vi "nanocal -- nuclear schottky fit -- 2x2 -- V9.vi"() -> ()   [LabVIEW 2021] (continued)
0.149623565609 ,     0.141877858801 } , \r{    0.018836490895 ,     0.149623565609 ,     0.115522422306 } , \r{    0.022387211386 ,     0.149623565609 ,     0.093179863408 } , \r{    0.026607250598 ,     0.149623565609 ,     0.074729843493 } , \r{    0.031622776602 ,     0.149623565609 ,     0.059995877610 } , \r{    0.037583740429 ,     0.149623565609 ,     0.048775938318 } , \r{    0.044668359215 ,     0.149623565609 ,     0.040874020839 } , \r{    0.053088444423 ,     0.149623565609 ,     0.036127045463 } , \r{    0.063095734448 ,     0.149623565609 ,     0.034421884157 } , \r{    0.074989420933 ,     0.149623565609 ,     0.035699674200 } , \r{    0.089125093813 ,     0.149623565609 ,     0.039947569357 } , \r{    0.105925372518 ,     0.149623565609 ,     0.047180252600 } , \r{    0.125892541179 ,     0.149623565609 ,     0.057414385167 } , \r{    0.149623565609 ,     0.149623565609 ,     0.070639278795 } , \r{    0.177827941004 ,     0.149623565609 ,     0.086787357406 } , \r{    0.211348903984 ,     0.149623565609 ,     0.105708646760 } , \r{    0.251188643151 ,     0.149623565609 ,     0.127153912456 } , \r{    0.298538261892 ,     0.149623565609 ,     0.150770299518 } , \r{    0.354813389234 ,     0.149623565609 ,     0.176111225707 } , \r{    0.421696503429 ,     0.149623565609 ,     0.202659475022 } , \r{    0.501187233627 ,     0.149623565609 ,     0.229859851640 } , \r{    0.595662143529 ,     0.149623565609 ,     0.257156086913 } , \r{    0.707945784384 ,     0.149623565609 ,     0.284026281992 } , \r{    0.841395141645 ,     0.149623565609 ,     0.310012042831 } , \r{    0.001000000000 ,     0.177827941004 ,     0.740836835011 } , \r{    0.001188502227 ,     0.177827941004 ,     0.710329495354 } , \r{    0.001412537545 ,     0.177827941004 ,     0.677050447028 } , \r{    0.001678804018 ,     0.177827941004 ,     0.641106189632 } , \r{    0.001995262315 ,     0.177827941004 ,     0.602678568915 } , \r{    0.002371373706 ,     0.177827941004 ,     0.562039454503 } , \r{    0.002818382931 ,     0.177827941004 ,     0.519566808327 } , \r{    0.003349654392 ,     0.177827941004 ,     0.475755530109 } , \r{    0.003981071706 ,     0.177827941004 ,     0.431214355020 } , \r{    0.004731512590 ,     0.177827941004 ,     0.386642000254 } , \r{    0.005623413252 ,     0.177827941004 ,     0.342782601520 } , \r{    0.006683439176 ,     0.177827941004 ,     0.300369479723 } , \r{    0.007943282347 ,     0.177827941004 ,     0.260071698430 } , \r{    0.009440608763 ,     0.177827941004 ,     0.222455656817 } , \r{    0.011220184543 ,     0.177827941004 ,     0.187965930155 } , \r{    0.013335214322 ,     0.177827941004 ,     0.156921789373 } , \r{    0.015848931925 ,     0.177827941004 ,     0.129522861582 } , \r{    0.018836490895 ,     0.177827941004 ,     0.105859097961 } , \r{    0.022387211386 ,     0.177827941004 ,     0.085923590392 } , \r{    0.026607250598 ,     0.177827941004 ,     0.069629182896 } , \r{    0.031622776602 ,     0.177827941004 ,     0.056830202835 } , \r{    0.037583740429 ,     0.177827941004 ,     0.047349108968 } , \r{    0.044668359215 ,     0.177827941004 ,     0.041005320854 } , \r{    0.053088444423 ,     0.177827941004 ,     0.037641414898 } , \r{    0.063095734448 ,     0.177827941004 ,     0.037141549042 } , \r{    0.074989420933 ,     0.177827941004 ,     0.039438657457 } , \r{    0.089125093813 ,     0.177827941004 ,     0.044509677824 } , \r{    0.105925372518 ,     0.177827941004 ,     0.052360451062 } , \r{    0.125892541179 ,     0.177827941004 ,     0.063003162991 } , \r{    0.149623565609 ,     0.177827941004 ,     0.076429499384 } , \r{    0.177827941004 ,     0.177827941004 ,     0.092582860491 } , \r{    0.211348903984 ,     0.177827941004 ,     0.111333482638 } , \r{    0.251188643151 ,     0.177827941004 ,     0.132460756805 } , \r{    0.298538261892 ,     0.177827941004 ,     0.155646612919 } , \r{    0.354813389234 ,     0.177827941004 ,     0.180482156819 } , \r{    0.421696503429 ,     0.177827941004 ,     0.206487187930 } , \r{    0.501187233627 ,     0.177827941004 ,     0.233139638088 } , \r{    0.595662143529 ,     0.177827941004 ,     0.259910134828 } , \r{    0.707945784384 ,     0.177827941004 ,     0.286296242008 } , \r{    0.841395141645 ,     0.177827941004 ,     0.311851541843 } , \r{    0.001000000000 ,     0.211348903984 ,     0.658706462723 } , \r{    0.001188502227 ,     0.211348903984 ,     0.632229697281 } , \r{    0.001412537545 ,     0.211348903984 ,     0.603327363418 } , \r{    0.001678804018 ,     0.211348903984 ,     0.572087346120 } , \r{    0.001995262315 ,     0.211348903984 ,     0.538656633281 } , \r{    0.002371373706 ,     0.211348903984 ,     0.503252529375 } , \r{    0.002818382931 ,     0.211348903984 ,     0.466177332768 } , \r{    0.003349654392 ,     0.211348903984 ,     0.427831696047 } , \r{    0.003981071706 ,     0.211348903984 ,     0.388719014145 } , \r{    0.004731512590 ,     0.211348903984 ,     0.349433142339 } , \r{    0.005623413252 ,     0.211348903984 ,     0.310626218644 } , \r{    0.006683439176 ,     0.211348903984 ,     0.272961381709 } , \r{    0.007943282347 ,     0.211348903984 ,     0.237062250981 } , \r{    0.009440608763 ,     0.211348903984 ,     0.203472092487 } , \r{    0.011220184543 ,     0.211348903984 ,     0.172629846218 } , \r{    0.013335214322 ,     0.211348903984 ,     0.144862225297 } , \r{    0.015848931925 ,     0.211348903984 ,     0.120386368340 } , \r{    0.018836490895 ,     0.211348903984 ,     0.099317684423 } , \r{    0.022387211386 ,     0.211348903984 ,     0.081680417039 } , \r{    0.026607250598 ,     0.211348903984 ,     0.067421184763 } , \r{    0.031622776602 ,     0.211348903984 ,     0.056426796441 } , \r{    0.037583740429 ,     0.211348903984 ,     0.048546798094 } , \r{    0.044668359215 ,     0.211348903984 ,     0.043619100040 } , \r{    0.053088444423 ,     0.211348903984 ,     0.041494839043 } , \r{    0.063095734448 ,     0.211348903984 ,     0.042057671458 } , \r{    0.074989420933 ,     0.211348903984 ,     0.045233607293 } , \r{    0.089125093813 ,     0.211348903984 ,     0.050989777453 } , \r{    0.105925372518 ,     0.211348903984 ,     0.059322962241 } , \r{    0.125892541179 ,     0.211348903984 ,     0.070240293599 } , \r{    0.149623565609 ,     0.211348903984 ,     0.083735123682 } , \r{    0.177827941004 ,     0.211348903984 ,     0.099761216436 } , \r{    0.211348903984 ,     0.211348903984 ,     0.118208753852 } , \r{    0.251188643151 ,     0.211348903984 ,     0.138886076738 } , \r{    0.298538261892 ,     0.211348903984 ,     0.161510944813 } , \r{    0.354813389234 ,     0.211348903984 ,     0.185713860663 } , \r{    0.421696503429 ,     0.211348903984 ,     0.211053773929 } , \r{    0.501187233627 ,     0.211348903984 ,     0.237043967586 } , \r{    0.595662143529 ,     0.211348903984 ,     0.263183941094 } , \r{    0.707945784384 ,     0.211348903984 ,     0.288992188714 } , \r{    0.841395141645 ,     0.211348903984 ,     0.314035081981 } , \r{    0.001000000000 ,     0.251188643151 ,     0.583753974070 } , \r{    0.001188502227 ,     0.251188643151 ,     0.561057464983 } , \r{    0.001412537545 ,     0.251188643151 ,     0.536261953482 } , \r{    0.001678804018 ,     0.251188643151 ,     0.509441674684 } , \r{    0.001995262315 ,     0.251188643151 ,     0.480716417964 } , \r{    0.002371373706 ,     0.251188643151 ,     0.450258891242 } , \r{    0.002818382931 ,     0.251188643151 ,     0.418306756758 } , \r{    0.003349654392 ,     0.251188643151 ,     0.385176391666 } , \r{    0.003981071706 ,     0.251188643151 ,     0.351272300628 } , \r{    0.004731512590 ,     0.251188643151 ,     0.317084637215 } , \r{    0.005623413252 ,     0.251188643151 ,     0.283169393408 } , \r{    0.006683439176 ,     0.251188643151 ,     0.250111957470 } , \r{    0.007943282347 ,     0.251188643151 ,     0.218482233638 } , \r{    0.009440608763 ,     0.251188643151 ,     0.188793416013 } , \r{    0.011220184543 ,     0.251188643151 ,     0.161473822961 } , \r{    0.013335214322 ,     0.251188643151 ,     0.136854159170 } , \r{    0.015848931925 ,     0.251188643151 ,     0.115166529542 } , \r{    0.018836490895 ,     0.251188643151 ,     0.096549850207 } , \r{    0.022387211386 ,     0.251188643151 ,     0.081058241465 } , \r{    0.026607250598 ,     0.251188643151 ,     0.068671793768 } , \r{    0.031622776602 ,     0.251188643151 ,     0.059310729766 } , \r{    0.037583740429 ,     0.251188643151 ,     0.052853849353 } , \r{    0.044668359215 ,     0.251188643151 ,     0.049160578455 } , \r{    0.053088444423 ,     0.251188643151 ,     0.048093842246 } , \r{    0.063095734448 ,     0.251188643151 ,     0.049539555202 } , \r{    0.074989420933 ,     0.251188643151 ,     0.053418665177 } , \r{    0.089125093813 ,     0.251188643151 ,     0.059689373296 } , \r{    0.105925372518 ,     0.251188643151 ,     0.068339460616 } , \r{    0.125892541179 ,     0.251188643151 ,     0.079370510719 } , \r{    0.149623565609 ,     0.251188643151 ,     0.092776735099 } , \r{    0.177827941004 ,     0.251188643151 ,     0.108521376077 } , \r{    0.211348903984 ,     0.251188643151 ,     0.126513873499 } , \r{    0.251188643151 ,     0.251188643151 ,     0.146591332212 } , \r{    0.298538261892 ,     0.251188643151 ,     0.168507891467 } , \r{    0.354813389234 ,     0.251188643151 ,     0.191934786010 } , \r{    0.421696503429 ,     0.251188643151 ,     0.216472066639 } , \r{    0.501187233627 ,     0.251188643151 ,     0.241670603037 } , \r{    0.595662143529 ,     0.251188643151 ,     0.267060904339 } , \r{    0.707945784384 ,     0.251188643151 ,     0.292184101542 } , \r{    0.841395141645 ,     0.251188643151 ,     0.316620409071 } , \r{    0.001000000000 ,     0.298538261892 ,     0.517704935038 } , \r{    0.001188502227 ,     0.298538261892 ,     0.498483642507 } , \r{    0.001412537545 ,     0.298538261892 ,     0.477463151719 } , \r{    0.001678804018 ,     0.298538261892 ,     0.454708039811 } , \r{    0.001995262315 ,     0.298538261892 ,     0.430317916888 } , \r{    0.002371373706 ,     0.298538261892 ,     0.404430957044 } , \r{    0.002818382931 ,     0.298538261892 ,     0.377232485595 } , \r{    0.003349654392 ,     0.298538261892 ,     0.348967315706 } , \r{    0.003981071706 ,     0.298538261892 ,     0.319951559176 } , \r{    0.004731512590 ,     0.298538261892 ,     0.290577377217 } , \r{    0.005623413252 ,     0.298538261892 ,     0.261304285049 } , \r{    0.006683439176 ,     0.298538261892 ,     0.232634443257 } , \r{    0.007943282347 ,     0.298538261892 ,     0.205075982287 } , \r{    0.009440608763 ,     0.298538261892 ,     0.179104073008 } , \r{    0.011220184543 ,     0.298538261892 ,     0.155130036145 } , \r{    0.013335214322 ,     0.298538261892 ,     0.133483847148 } , \r{    0.015848931925 ,     0.298538261892 ,     0.114408951404 } , \r{    0.018836490895 ,     0.298538261892 ,     0.098064811086 } , \r{    0.022387211386 ,     0.298538261892 ,     0.084533116759 } , \r{    0.026607250598 ,     0.298538261892 ,     0.073826084038 } , \r{    0.031622776602 ,     0.298538261892 ,     0.065897330233 } , \r{    0.037583740429 ,     0.298538261892 ,     0.060656379298 } , \r{    0.044668359215 ,     0.298538261892 ,     0.057986900287 } , \r{    0.053088444423 ,     0.298538261892 ,     0.057766973425 } , \r{    0.063095734448 ,     0.298538261892 ,     0.059887999585 } , \r{    0.074989420933 ,     0.298538261892 ,     0.064268325763 } , \r{    0.089125093813 ,     0.298538261892 ,     0.070858633213 } , \r{    0.105925372518 ,     0.298538261892 ,     0.079638111104 } , \r{    0.125892541179 ,     0.298538261892 ,     0.090602425808 } , \r{    0.149623565609 ,     0.298538261892 ,     0.103745757535 } , \r{    0.177827941004 ,     0.298538261892 ,     0.119039662023 } , \r{    0.211348903984 ,     0.298538261892 ,     0.136411689542 } , \r{    0.251188643151 ,     0.298538261892 ,     0.155726935779 } , \r{    0.298538261892 ,     0.298538261892 ,     0.176775860178 } , \r{    0.354813389234 ,     0.298538261892 ,     0.199271268192 } , \r{    0.421696503429 ,     0.298538261892 ,     0.222855986016 } , \r{    0.501187233627 ,     0.298538261892 ,     0.247120689274 } , \r{    0.595662143529 ,     0.298538261892 ,     0.271629244883 } , \r{    0.707945784384 ,     0.298538261892 ,     0.295947480550 } , \r{    0.841395141645 ,     0.298538261892 ,     0.319670904915 } , \r{    0.001000000000 ,     0.354813389234 ,     0.461802046903 } , \r{    0.001188502227 ,     0.354813389234 ,     0.445715861517 } , \r{    0.001412537545 ,     0.354813389234 ,     0.428098537544 } , \r{    0.001678804018 ,     0.354813389234 ,     0.409007654015 } , \r{    0.001995262315 ,     0.354813389234 ,     0.388528341511 } , \r{    0.002371373706 ,     0.354813389234 ,     0.366773369859 } , \r{    0.002818382931 ,     0.354813389234 ,     0.343887989903 } , \r{    0.003349654392 ,     0.354813389234 ,     0.320059548601 } , \r{    0.003981071706 ,     0.354813389234 ,     0.295529331319 } , \r{    0.004731512590 ,     0.354813389234 ,     0.270601601307 } , \r{    0.005623413252 ,     0.354813389234 ,     0.245643669355 } , \r{    0.006683439176 ,     0.354813389234 ,     0.221072447582 } , \r{    0.007943282347 ,     0.354813389234 ,     0.197327737812 } , \r{    0.009440608763 ,     0.354813389234 ,     0.174838486318 } , \r{    0.011220184543 ,     0.354813389234 ,     0.153991480792 } , \r{    0.013335214322 ,     0.354813389234 ,     0.135109942669 } , \r{    0.015848931925 ,     0.354813389234 ,     0.118443882956 } , \r{    0.018836490895 ,     0.354813389234 ,     0.104169302093 } , \r{    0.022387211386 ,     0.354813389234 ,     0.092392082586 } , \r{    0.026607250598 ,     0.354813389234 ,     0.083154079639 } , \r{    0.031622776602 ,     0.354813389234 ,     0.076441152816 } , \r{    0.037583740429 ,     0.354813389234 ,     0.072194056197 } , \r{    0.044668359215 ,     0.354813389234 ,     0.070322824798 } , \r{    0.053088444423 ,     0.354813389234 ,     0.070723930547 } , \r{    0.063095734448 ,     0.354813389234 ,     0.073297794987 } , \r{    0.074989420933 ,     0.354813389234 ,     0.077963185268 } , \r{    0.089125093813 ,     0.354813389234 ,     0.084665252670 } , \r{    0.105925372518 ,     0.354813389234 ,     0.093375422231 } , \r{    0.125892541179 ,     0.354813389234 ,     0.104083257620 } , \r{    0.149623565609 ,     0.354813389234 ,     0.116781962397 } , \r{    0.177827941004 ,     0.354813389234 ,     0.131449965768 } , \r{    0.211348903984 ,     0.354813389234 ,     0.148031298487 } , \r{    0.251188643151 ,     0.354813389234 ,     0.166417619532 } , \r{    0.298538261892 ,     0.354813389234 ,     0.186434918726 } , \r{    0.354813389234 ,     0.354813389234 ,     0.207837754480 } , \r{    0.421696503429 ,     0.354813389234 ,     0.230312971944 } , \r{    0.501187233627 ,     0.354813389234 ,     0.253493157225 } , \r{    0.595662143529 ,     0.354813389234 ,     0.276978084046 } , \r{    0.707945784384 ,     0.354813389234 ,     0.300360774991 } , \r{    0.841395141645 ,     0.354813389234 ,     0.323254041024 } , \r{    0.001000000000 ,     0.421696503429 ,     0.416711745146 } , \r{    0.001188502227 ,     0.421696503429 ,     0.403405424373 } , \r{    0.001412537545 ,     0.421696503429 ,     0.388801996550 } , \r{    0.001678804018 ,     0.421696503429 ,     0.372953265916 } , \r{    0.001995262315 ,     0.421696503429 ,     0.355933853019 } , \r{    0.002371373706 ,     0.421696503429 ,     0.337838521448 } , \r{    0.002818382931 ,     0.421696503429 ,     0.318783451795 } , \r{    0.003349654392 ,     0.421696503429 ,     0.298912458920 } , \r{    0.003981071706 ,     0.421696503429 ,     0.278407081902 } , \r{    0.004731512590 ,     0.421696503429 ,     0.257497137785 } , \r{    0.005623413252 ,     0.421696503429 ,     0.236466581026 } , \r{    0.006683439176 ,     0.421696503429 ,     0.215649499411 } , \r{    0.007943282347 ,     0.421696503429 ,     0.195413771552 } , \r{    0.009440608763 ,     0.421696503429 ,     0.176134888784 } , \r{    0.011220184543 ,     0.421696503429 ,     0.158167059297 } , \r{    0.013335214322 ,     0.421696503429 ,     0.141819622963 } , \r{    0.015848931925 ,     0.421696503429 ,     0.127343271395 } , \r{    0.018836490895 ,     0.421696503429 ,     0.114925528459 } , \r{    0.022387211386 ,     0.421696503429 ,     0.104692064238 } , \r{    0.026607250598 ,     0.421696503429 ,     0.096710743330 } , \r{    0.031622776602 ,     0.421696503429 ,     0.090997273470 } , \r{    0.037583740429 ,     0.421696503429 ,     0.087522948802 } , \r{    0.044668359215 ,     0.421696503429 ,     0.086225360489 } , \r{    0.053088444423 ,     0.421696503429 ,     0.087022135267 } , \r{    0.063095734448 ,     0.421696503429 ,     0.089826294113 } , \r{    0.074989420933 ,     0.421696503429 ,     0.094560484261 } , \r{    0.089125093813 ,     0.421696503429 ,     0.101166907408 } , \r{    0.105925372518 ,     0.421696503429 ,     0.109610554380 } , \r{    0.125892541179 ,     0.421696503429 ,     0.119874971535 } , \r{    0.149623565609 ,     0.421696503429 ,     0.131951445202 } , \r{    0.177827941004 ,     0.421696503429 ,     0.145823593529 } , \r{    0.211348903984 ,     0.421696503429 ,     0.161449818861 } , \r{    0.251188643151 ,     0.421696503429 ,     0.178746221763 } , \r{    0.298538261892 ,     0.421696503429 ,     0.197572693944 } , \r{    0.354813389234 ,     0.421696503429 ,     0.217724892271 } , \r{    0.421696503429 ,     0.421696503429 ,     0.238934275633 } , \r{    0.501187233627 ,     0.421696503429 ,     0.260877135971 } , \r{    0.595662143529 ,     0.421696503429 ,     0.283191791372 } , \r{    0.707945784384 ,     0.421696503429 ,     0.305501396843 } , \r{    0.841395141645 ,     0.421696503429 ,     0.327438742692 } , \r{    0.001000000000 ,     0.501187233627 ,     0.382498963678 } , \r{    0.001188502227 ,     0.501187233627 ,     0.371619717619 } , \r{    0.001412537545 ,     0.501187233627 ,     0.359643822955 } , \r{    0.001678804018 ,     0.501187233627 ,     0.346617257902 } , \r{    0.001995262315 ,     0.501187233627 ,     0.332606289949 } , \r{    0.002371373706 ,     0.501187233627 ,     0.317692910823 } , \r{    0.002818382931 ,     0.501187233627 ,     0.301973094158 } , \r{    0.003349654392 ,     0.501187233627 ,     0.285559516092 } , \r{    0.003981071706 ,     0.501187233627 ,     0.268588823278 } , \r{    0.004731512590 ,     0.501187233627 ,     0.251231514228 } , \r{    0.005623413252 ,     0.501187233627 ,     0.233700619039 } , \r{    0.006683439176 ,     0.501187233627 ,     0.216254420067 } , \r{    0.007943282347 ,     0.501187233627 ,     0.199189383598 } , \r{    0.009440608763 ,     0.501187233627 ,     0.182822738472 } , \r{    0.011220184543 ,     0.501187233627 ,     0.167468647881 } , \r{    0.013335214322 ,     0.501187233627 ,     0.153414887674 } , \r{    0.015848931925 ,     0.501187233627 ,     0.140906053700 } , \r{    0.018836490895 ,     0.501187233627 ,     0.130135312395 } , \r{    0.022387211386 ,     0.501187233627 ,     0.121242839483 } , \r{    0.026607250598 ,     0.501187233627 ,     0.114317848157 } , \r{    0.031622776602 ,     0.501187233627 ,     0.109402268895 } , \r{    0.037583740429 ,     0.501187233627 ,     0.106495908924 } , \r{    0.044668359215 ,     0.501187233627 ,     0.105563878676 } , \r{    0.053088444423 ,     0.501187233627 ,     0.106546864479 } , \r{    0.063095734448 ,     0.501187233627 ,     0.109373749657 } , \r{    0.074989420933 ,     0.501187233627 ,     0.113974731139 } , \r{    0.089125093813 ,     0.501187233627 ,     0.120292172945 } , \r{    0.105925372518 ,     0.501187233627 ,     0.128286535662 } , \r{    0.125892541179 ,     0.501187233627 ,     0.137935828301 } , \r{    0.149623565609 ,     0.501187233627 ,     0.149228595672 } , \r{    0.177827941004 ,     0.501187233627 ,     0.162151793987 } , \r{    0.211348903984 ,     0.501187233627 ,     0.176675657566 } , \r{    0.251188643151 ,     0.501187233627 ,     0.192737921294 } , \r{    0.298538261892 ,     0.501187233627 ,     0.210229847437 } , \r{    0.354813389234 ,     0.501187233627 ,     0.228986534293 } , \r{    0.421696503429 ,     0.501187233627 ,     0.248783743287 } , \r{    0.501187233627 ,     0.501187233627 ,     0.269342666886 } , \r{    0.595662143529 ,     0.501187233627 ,     0.290342647138 } , \r{    0.707945784384 ,     0.501187233627 ,     0.311440212229 } , \r{    0.841395141645 ,     0.501187233627 ,     0.332291480224 } , \r{    0.001000000000 ,     0.595662143529 ,     0.358671219729 } , \r{    0.001188502227 ,     0.595662143529 ,     0.349882157487 } , \r{    0.001412537545 ,     0.595662143529 ,     0.340166106960 } , \r{    0.001678804018 ,     0.595662143529 ,     0.329562278481 } , \r{    0.001995262315 ,     0.595662143529 ,     0.318129160990 } , \r{    0.002371373706 ,     0.595662143529 ,     0.305939009622 } , \r{    0.002818382931 ,     0.595662143529 ,     0.293073891561 } , \r{    0.003349654392 ,     0.595662143529 ,     0.279625268208 } , \r{    0.003981071706 ,     0.595662143529 ,     0.265698037639 } , \r{    0.004731512590 ,     0.595662143529 ,     0.251418323562 } , \r{    0.005623413252 ,     0.595662143529 ,     0.236942532027 } , \r{    0.006683439176 ,     0.595662143529 ,     0.222463874544 } , \r{    0.007943282347 ,     0.595662143529 ,     0.208212349848 } , \r{    0.009440608763 ,     0.595662143529 ,     0.194445756283 } , \r{    0.011220184543 ,     0.595662143529 ,     0.181432674722 } , \r{    0.013335214322 ,     0.595662143529 ,     0.169432005561 } , \r{    0.015848931925 ,     0.595662143529 ,     0.158675053766 } , \r{    0.018836490895 ,     0.595662143529 ,     0.149354151962 } , \r{    0.022387211386 ,     0.595662143529 ,     0.141618074195 } , \r{    0.026607250598 ,     0.595662143529 ,     0.135571936594 } , \r{    0.031622776602 ,     0.595662143529 ,     0.131279200532 } , \r{    0.037583740429 ,     0.595662143529 ,     0.128764831083 } , \r{    0.044668359215 ,     0.595662143529 ,     0.128020006149 } , \r{    0.053088444423 ,     0.595662143529 ,     0.129009158286 } , \r{    0.063095734448 ,     0.595662143529 ,     0.131679552968 } , \r{    0.074989420933 ,     0.595662143529 ,     0.135972465039 } , \r{    0.089125093813 ,     0.595662143529 ,     0.141833892977 } , \r{    0.105925372518 ,     0.595662143529 ,     0.149222265177 } , \r{    0.125892541179 ,     0.595662143529 ,     0.158111070502 } , \r{    0.149623565609 ,     0.595662143529 ,     0.168485578802 } , \r{    0.177827941004 ,     0.595662143529 ,     0.180334217329 } , \r{    0.211348903984 ,     0.595662143529 ,     0.193636197284 } , \r{    0.251188643151 ,     0.595662143529 ,     0.208347473588 } , \r{    0.298538261892 ,     0.595662143529 ,     0.224387257855 } , \r{    0.354813389234 ,     0.595662143529 ,     0.241627329089 } , \r{    0.421696503429 ,     0.595662143529 ,     0.259886293333 } , \r{    0.501187233627 ,     0.595662143529 ,     0.278930488434 } , \r{    0.595662143529 ,     0.595662143529 ,     0.298482226423 } , \r{    0.707945784384 ,     0.595662143529 ,     0.318234646419 } , \r{    0.841395141645 ,     0.595662143529 ,     0.337871047210 } , \r{    0.001000000000 ,     0.707945784384 ,     0.344279898358 } , \r{    0.001188502227 ,     0.707945784384 ,     0.337268699566 } , \r{    0.001412537545 ,     0.707945784384 ,     0.329473699264 } , \r{    0.001678804018 ,     0.707945784384 ,     0.320926024993 } , \r{    0.001995262315 ,     0.707945784384 ,     0.311675849778 } , \r{    0.002371373706 ,     0.707945784384 ,     0.301786837397 } , \r{    0.002818382931 ,     0.707945784384 ,     0.291330912344 } , \r{    0.003349654392 ,     0.707945784384 ,     0.280385385593 } , \r{    0.003981071706 ,     0.707945784384 ,     0.269033897700 } , \r{    0.004731512590 ,     0.707945784384 ,     0.257371418611 } , \r{    0.005623413252 ,     0.707945784384 ,     0.245512000288 } , \r{    0.006683439176 ,     0.707945784384 ,     0.233596579236 } , \r{    0.007943282347 ,     0.707945784384 ,     0.221797353004 } , \r{    0.009440608763 ,     0.707945784384 ,     0.210315629843 } , \r{    0.011220184543 ,     0.707945784384 ,     0.199371982981 } , \r{    0.013335214322 ,     0.707945784384 ,     0.189190656542 } , \r{    0.015848931925 ,     0.707945784384 ,     0.179982798322 } , \r{    0.018836490895 ,     0.707945784384 ,     0.171933260980 } , \r{    0.022387211386 ,     0.707945784384 ,     0.165193225134 } , \r{    0.026607250598 ,     0.707945784384 ,     0.159877837071 } , \r{    0.031622776602 ,     0.707945784384 ,     0.156066657041 } , \r{    0.037583740429 ,     0.707945784384 ,     0.153805323136 } , \r{    0.044668359215 ,     0.707945784384 ,     0.153108205787 } , \r{    0.053088444423 ,     0.707945784384 ,     0.153962709019 } , \r{    0.063095734448 ,     0.707945784384 ,     0.156335838322 } , \r{    0.074989420933 ,     0.707945784384 ,     0.160182884907 } , \r{    0.089125093813 ,     0.707945784384 ,     0.165456998590 } , \r{    0.105925372518 ,     0.707945784384 ,     0.172117574384 } , \r{    0.125892541179 ,     0.707945784384 ,     0.180135244398 } , \r{    0.149623565609 ,     0.707945784384 ,     0.189491979043 } , \r{    0.177827941004 ,     0.707945784384 ,     0.200176026648 } , \r{    0.211348903984 ,     0.707945784384 ,     0.212172607819 } , \r{    0.251188643151 ,     0.707945784384 ,     0.225452043162 } , \r{    0.298538261892 ,     0.707945784384 ,     0.239957297520 } , \r{    0.354813389234 ,     0.707945784384 ,     0.255592977770 } , \r{    0.421696503429 ,     0.707945784384 ,     0.272217779186 } , \r{    0.501187233627 ,     0.707945784384 ,     0.289642152560 } , \r{    0.595662143529 ,     0.707945784384 ,     0.307632344406 } , \r{    0.707945784384 ,     0.707945784384 ,     0.325920877303 } , \r{    0.841395141645 ,     0.707945784384 ,     0.344222221305 } , \r{    0.001000000000 ,     0.841395141645 ,     0.338057235803 } , \r{    0.001188502227 ,     0.841395141645 ,     0.332540491283 } , \r{    0.001412537545 ,     0.841395141645 ,     0.326361600129 } , \r{    0.001678804018 ,     0.841395141645 ,     0.319542452651 } , \r{    0.001995262315 ,     0.841395141645 ,     0.312123858442 } , \r{    0.002371373706 ,     0.841395141645 ,     0.304160702070 } , \r{    0.002818382931 ,     0.841395141645 ,     0.295716376983 } , \r{    0.003349654392 ,     0.841395141645 ,     0.286858333364 } , \r{    0.003981071706 ,     0.841395141645 ,     0.277656438145 } , \r{    0.004731512590 ,     0.841395141645 ,     0.268185069466 } , \r{    0.005623413252 ,     0.841395141645 ,     0.258528621406 } , \r{    0.006683439176 ,     0.841395141645 ,     0.248788759073 } , \r{    0.007943282347 ,     0.841395141645 ,     0.239090758823 } , \r{    0.009440608763 ,     0.841395141645 ,     0.229585965790 } , \r{    0.011220184543 ,     0.841395141645 ,     0.220448175740 } , \r{    0.013335214322 ,     0.841395141645 ,     0.211863777840 } , \r{    0.015848931925 ,     0.841395141645 ,     0.204018144929 } , \r{    0.018836490895 ,     0.841395141645 ,     0.197082412434 } , \r{    0.022387211386 ,     0.841395141645 ,     0.191204095814 } , \r{    0.026607250598 ,     0.841395141645 ,     0.186502488296 } , \r{    0.031622776602 ,     0.841395141645 ,     0.183067526296 } , \r{    0.037583740429 ,     0.841395141645 ,     0.180960295139 } , \r{    0.044668359215 ,     0.841395141645 ,     0.180214276074 } , \r{    0.053088444423 ,     0.841395141645 ,     0.180837571382 } , \r{    0.063095734448 ,     0.841395141645 ,     0.182816821978 } , \r{    0.074989420933 ,     0.841395141645 ,     0.186123219061 } , \r{    0.089125093813 ,     0.841395141645 ,     0.190720178045 } , \r{    0.105925372518 ,     0.841395141645 ,     0.196571299937 } , \r{    0.125892541179 ,     0.841395141645 ,     0.203646663557 } , \r{    0.149623565609 ,     0.841395141645 ,     0.211925622011 } , \r{    0.177827941004 ,     0.841395141645 ,     0.221395103699 } , \r{    0.211348903984 ,     0.841395141645 ,     0.232043555101 } , \r{    0.251188643151 ,     0.841395141645 ,     0.243851634664 } , \r{    0.298538261892 ,     0.841395141645 ,     0.256781317268 } , \r{    0.354813389234 ,     0.841395141645 ,     0.270765245362 } , \r{    0.421696503429 ,     0.841395141645 ,     0.285698155030 } , \r{    0.501187233627 ,     0.841395141645 ,     0.301432093581 } , \r{    0.595662143529 ,     0.841395141645 ,     0.317776809420 } , \r{    0.707945784384 ,     0.841395141645 ,     0.334505973391 } , \r{    0.841395141645 ,     0.841395141645 ,     0.351368812895 } , \r }   "
  out "cursor x selector":map{T2, dbl}(c390)
  in  ":sweep is ON":bool
  in  "win":T16={"cen (Hz)"=23772.179970264126, "win (Hz)"=4484.832860239923, "left (Hz)"=21529.763540144166, "right (Hz)"=26014.596400384085}
  in  "cursor window":T17={"left"=20184.313682072192, "right "=24669.14654231211, "center"=22426.730112192152, "window"=4484.832860239923, "cursors"=[0, 1, 2], "relative"=0, "absolute"=0, "fixed vertical offset"=0.0, "vertical offset"=0.0, "skew"=0.0, "default window frac"=0.1, "kind"=enum."symmetric", "skew.left"=0.5, "skew.right"=0.5, "Plot ref"=refnum, "wing order"=enum."forw"}
  out "color data":cluster{"Array":dbl[], "Array":dbl[]}[](array[cluster])=[{"Array"=[0.12, 0.148, 0.15, 0.17, 0.2, 0.25, 0.3, 0.36, 0.42, 0.52, 0.62, 0.82, 1.12, 1.7, 1.9, 3.1, 5.7], "Array"=[0.62728998582, 0.2730109012575849, 0.4360358231158382, 0.31273882707493267, 0.21185679953244455, 0.14497429295634315, 0.10320507255338958, 0.06738649827292763, 0.022507492936216303, 0.021849716434935364, 0.021729475893381252, 0.0198519726342436, 0.016283381951146165, 0.01886089700009046, 0.017534515105553365, 0.01657901647493233, 0.017491792324152208]}, {"Array"=[0.12, 0.148, 0.15, 0.17, 0.2, 0.25, 0.3, 0.36, 0.42, 0.52, 0.62, 0.82, 1.12, 1.7, 1.9, 3.1, 5.7], "Array"=[0.23974349678, 0.07091543775458298, 0.13629832485566626, 0.15316677568416495, 0.17371303124805412, 0.27815367910908206, 0.4568771678095196, 0.03375938315839582, 0.03387143424300576, 0.033883152649051125, 0.03390178634313435, 0.03384656153160249, 0.03390452446017073, 0.03378369231014688, 0.02323861783817173, 0.029207680038740087, 0.02587551529326107]}, {"Array"=[0.12, 0.148, 0.15, 0.17, 0.2, 0.25, 0.3, 0.36, 0.42, 0.52, 0.62, 0.82, 1.12, 1.7, 1.9, 3.1, 5.7], "Array"=[0.076926495749, 0.13557684408337248, 0.03542880244691447, 0.02942840377205427, 0.02504707721851352, 0.020087180736490247, 0.018190810679879554, 0.0163524675075112, 0.016835987172777216, 0.01819702773822382, 0.020153498516221252, 0.023547995635674095, 0.031661688913314306, 0.03349591654527996, 0.014265591932458873, 0.009191722708188048, 0.005854448603805341]}, {"Array"=[0.12, 0.148, 0.15, 0.17, 0.2, 0.25, 0.3, 0.36, 0.42, 0.52, 0.62, 0.82, 1.12, 1.7, 1.9, 3.1, 5.7], "Array"=[0.159415903746, 0.04012911681217574, 0.042141009445427945, 0.032059842594624494, 0.02279985029361622, 0.018878235168909133, 0.020353539568818982, 5.5602042137039274e-05, 0.00021346840235837033, 0.00021340250099372794, 0.00021321792059620005, 0.00027413175252649695, 0.0002745370162211529, 0.0004261574975821111, 0.000383027800546881, 0.0002822141564676873, 0.00033678261197217014]}, {"Array"=[0.12, 0.148, 0.15, 0.17, 0.2, 0.25, 0.3, 0.36, 0.42, 0.52, 0.62, 0.82, 1.12, 1.7, 1.9, 3.1, 5.7], "Array"=[0.000763641667, 0.0009923872987074498, 0.0008634344957269274, 0.000966119229084584, 0.0011194877919145127, 0.0013606502621125451, 0.0015326336783234693, 0.002052818741953473, 0.0017781658353584764, 0.001801850307392029, 0.0018089734240976446, 0.002984103948241005, 0.003250738484609814, 0.0031602960429135524, 0.002949269667352954, 0.002421267656945163, 0.002022629565026247]}, {"Array"=[0.12, 0.148, 0.15, 0.17, 0.2, 0.25, 0.3, 0.36, 0.42, 0.52, 0.62, 0.82, 1.12, 1.7, 1.9, 3.1, 5.7], "Array"=[4.35e-10, 6.439381253023805e-10, 6.308810838918409e-10, 7.625114350763984e-10, 8.195852207774218e-10, 1.2510608054547487e-09, 1.5572561005318226e-09, 2.053450896656566e-09, 2.479707154238972e-09, 3.1313474594286157e-09, 3.806148532350378e-09, 5.213755545903577e-09, 7.2628137959888106e-09, 1.1406421503525573e-08, 1.2895431292182517e-08, 2.227660928974633e-08, 5.4777678949124484e-08]}, {"Array"=[0.12, 0.148, 0.15, 0.17, 0.2, 0.25, 0.3, 0.36, 0.42, 0.52, 0.62, 0.82, 1.12, 1.7, 1.9, 3.1, 5.7], "Array"=[0.245568364347, 0.0645900574929368, 0.08004705050622966, 0.19487148720579237, 0.03351434142711687, 0.02184431417017586, 0.032347659490051216, 0.002480419109659059, 0.007814821925534395, 0.00520013588180238, 0.006296094438005391, 0.001908169809423058, 0.002257620140211018, 0.008605835968785608, 0.0024989962580555026, 0.003215464238537897, 0.003570816055454911]}, {"Array"=[0.12, 0.148, 0.15, 0.17, 0.2, 0.25, 0.3, 0.36, 0.42, 0.52, 0.62, 0.82, 1.12, 1.7, 1.9, 3.1, 5.7], "Array"=[0.022170590915, 0.01641248298202389, 0.002312030386804106, 0.0014819318949486784, 0.00035662888776441895, 0.00015894172062156444, 0.00010225804136915292, 0.0001282920284827463, 0.0003857404741353476, 0.00019678175234393364, 0.0002692480741424916, 0.00013393087590862188, 0.00016283980709594313, 0.00045778261364612133, 0.0003120318371061343, 8.8801730217525e-05, 7.291236500401702e-05]}, {"Array"=[0.12, 0.148, 0.15, 0.17, 0.2, 0.25, 0.3, 0.36, 0.42, 0.52, 0.62, 0.82, 1.12, 1.7, 1.9, 3.1, 5.7], "Array"=[0.126655465898, 0.016122106455977173, 0.019370507574418105, 0.032515587695104, 0.003953255270019443, 0.0013746091281296251, 0.0011727018719404464, 1.3396144617265272e-06, 1.8309382419984372e-05, 1.6694885155659994e-05, 1.6264646942714422e-05, 2.638451785235589e-06, 9.699549898748168e-06, 7.027190427402306e-05, 9.499625775806485e-06, 1.529926658584193e-05, 2.3576375004937536e-05]}]
  out "R(ω) fit out":cdb[](array[numeric])
  in  "parameter map":map{T2, dbl}(c390)
  out "filesnames lookup":map{i32, string}(c390)={0="IDS0183_210310_RAW_cal__sam_", 1="IDS0311_210901_RAW_cal__sam_", 2="IDS0359_210907_RAW_cal__sam_", 3="IDS0412_220525_RAW_cal__sam_", 4="IDS0431_220527_RAW_cal__sam_", 5="IDS0442_220528_RAW_cal__sam_", 6="IDS0464_220530_RAW_cal__sam_", 7="IDS0486_220602_RAW_cal__sam_", 8="IDS0336_210904_RAW_cal__sam_", 9="IDS0346_210904_RAW_cal__sam_", 10="IDS0378_210909_RAW_cal__sam_", 11="IDS0158_210310_RAW_cal__sam_", 12="IDS0300_210427_RAW_cal__sam_", 13="IDS0184_210310_RAW_cal__sam_", 14="IDS0210_210310_RAW_cal__sam_", 15="IDS0379_210909_RAW_cal__sam_", 16="IDS0360_210907_RAW_cal__sam_", 17="IDS0411_220525_RAW_cal__sam_", 18="IDS0427_220526_RAW_cal__sam_", 19="IDS0443_220528_RAW_cal__sam_", 20="IDS0463_220530_RAW_cal__sam_", 21="IDS0487_220602_RAW_cal__sam_", 22="IDS0310_210901_RAW_cal__sam_", 23="IDS0337_210904_RAW_cal__sam_", 24="IDS0347_210906_RAW_cal__sam_", 25="IDS0305_210831_RAW_cal__sam_", 26="IDS0361_210908_RAW_cal__sam_", 27="IDS0380_210909_RAW_cal__sam_", 28="IDS0159_210310_RAW_cal__sam_", 29="IDS0304_210831_RAW_cal__sam_", 30="IDS0312_210901_RAW_cal__sam_", 31="IDS0338_210904_RAW_cal__sam_", 32="IDS0410_220525_RAW_cal__sam_", 33="IDS0432_220527_RAW_cal__sam_", 34="IDS0444_220528_RAW_cal__sam_", 35="IDS0462_220530_RAW_cal__sam_", 36="IDS0485_220601_RAW_cal__sam_", 37="IDS0348_210906_RAW_cal__sam_", 38="IDS0181_210310_RAW_cal__sam_", 39="IDS0424_220526_RAW_cal__sam_", 40="IDS0185_210310_RAW_cal__sam_", 41="IDS0208_210310_RAW_cal__sam_", 42="IDS0209_210310_RAW_cal__sam_", 43="IDS0211_210310_RAW_cal__sam_", 44="IDS0212_210310_RAW_cal__sam_", 45="IDS0213_210310_RAW_cal__sam_", 46="IDS0214_210310_RAW_cal__sam_", 47="IDS0215_210310_RAW_cal__sam_", 48="IDS0216_210310_RAW_cal__sam_", 49="IDS0217_210310_RAW_cal__sam_", 50="IDS0330_210901_RAW_cal__sam_", 51="IDS0331_210901_RAW_cal__sam_", 52="IDS0335_210904_RAW_cal__sam_", 53="IDS0362_210908_RAW_cal__sam_", 54="IDS0377_210909_RAW_cal__sam_", 55="IDS0160_210310_RAW_cal__sam_", 56="IDS0303_210831_RAW_cal__sam_", 57="IDS0313_210901_RAW_cal__sam_", 58="IDS0349_210906_RAW_cal__sam_", 59="IDS0407_220525_RAW_cal__sam_", 60="IDS0441_220527_RAW_cal__sam_", 61="IDS0458_220529_RAW_cal__sam_", 62="IDS0477_220601_RAW_cal__sam_", 63="IDS0161_210310_RAW_cal__sam_", 64="IDS0186_210310_RAW_cal__sam_", 65="IDS0302_210831_RAW_cal__sam_", 66="IDS0363_210908_RAW_cal__sam_", 67="IDS0381_210909_RAW_cal__sam_", 68="IDS0408_220525_RAW_cal__sam_", 69="IDS0425_220526_RAW_cal__sam_", 70="IDS0445_220528_RAW_cal__sam_", 71="IDS0459_220529_RAW_cal__sam_", 72="IDS0478_220601_RAW_cal__sam_", 73="IDS0314_210901_RAW_cal__sam_", 74="IDS0339_210904_RAW_cal__sam_", 75="IDS0350_210906_RAW_cal__sam_", 76="IDS0162_210310_RAW_cal__sam_", 77="IDS0187_210310_RAW_cal__sam_", 78="IDS0301_210831_RAW_cal__sam_", 79="IDS0315_210901_RAW_cal__sam_", 80="IDS0382_210909_RAW_cal__sam_", 81="IDS0409_220525_RAW_cal__sam_", 82="IDS0426_220526_RAW_cal__sam_", 83="IDS0446_220528_RAW_cal__sam_", 84="IDS0460_220529_RAW_cal__sam_", 85="IDS0479_220601_RAW_cal__sam_", 86="IDS0364_210908_RAW_cal__sam_", 87="IDS0340_210904_RAW_cal__sam_", 88="IDS0351_210906_RAW_cal__sam_", 89="IDS0163_210310_RAW_cal__sam_", 90="IDS0188_210310_RAW_cal__sam_", 91="IDS0299_210427_RAW_cal__sam_", 92="IDS0316_210901_RAW_cal__sam_", 93="IDS0341_210904_RAW_cal__sam_", 94="IDS0352_210906_RAW_cal__sam_", 95="IDS0365_210908_RAW_cal__sam_", 96="IDS0383_210910_RAW_cal__sam_", 97="IDS0413_220525_RAW_cal__sam_", 98="IDS0428_220526_RAW_cal__sam_", 99="IDS0447_220528_RAW_cal__sam_", 100="IDS0461_220529_RAW_cal__sam_", 101="IDS0480_220601_RAW_cal__sam_", 102="IDS0164_210310_RAW_cal__sam_", 103="IDS0429_220526_RAW_cal__sam_", 104="IDS0448_220528_RAW_cal__sam_", 105="IDS0481_220601_RAW_cal__sam_", 106="IDS0189_210310_RAW_cal__sam_", 107="IDS0298_210427_RAW_cal__sam_", 108="IDS0317_210901_RAW_cal__sam_", 109="IDS0366_210908_RAW_cal__sam_", 110="IDS0384_210910_RAW_cal__sam_", 111="IDS0414_220525_RAW_cal__sam_", 112="IDS0465_220530_RAW_cal__sam_", 113="IDS0342_210904_RAW_cal__sam_", 114="IDS0353_210906_RAW_cal__sam_", 115="IDS0165_210310_RAW_cal__sam_", 116="IDS0190_210310_RAW_cal__sam_", 117="IDS0430_220526_RAW_cal__sam_", 118="IDS0449_220528_RAW_cal__sam_", 119="IDS0482_220601_RAW_cal__sam_", 120="IDS0297_210427_RAW_cal__sam_", 121="IDS0318_210901_RAW_cal__sam_", 122="IDS0343_210904_RAW_cal__sam_", 123="IDS0354_210906_RAW_cal__sam_", 124="IDS0367_210908_RAW_cal__sam_", 125="IDS0385_210910_RAW_cal__sam_", 126="IDS0415_220525_RAW_cal__sam_", 127="IDS0466_220530_RAW_cal__sam_", 128="IDS0166_210310_RAW_cal__sam_", 129="IDS0191_210310_RAW_cal__sam_", 130="IDS0296_210427_RAW_cal__sam_", 131="IDS0319_210901_RAW_cal__sam_", 132="IDS0344_210904_RAW_cal__sam_", 133="IDS0433_220527_RAW_cal__sam_", 134="IDS0450_220528_RAW_cal__sam_", 135="IDS0467_220530_RAW_cal__sam_", 136="IDS0483_220601_RAW_cal__sam_", 137="IDS0368_210908_RAW_cal__sam_", 138="IDS0386_210910_RAW_cal__sam_", 139="IDS0416_220525_RAW_cal__sam_", 140="IDS0220_210310_RAW_cal__sam_", 141="IDS0167_210310_RAW_cal__sam_", 142="IDS0192_210310_RAW_cal__sam_", 143="IDS0434_220527_RAW_cal__sam_", 144="IDS0451_220528_RAW_cal__sam_", 145="IDS0468_220530_RAW_cal__sam_", 146="IDS0484_220601_RAW_cal__sam_", 147="IDS0295_210427_RAW_cal__sam_", 148="IDS0320_210901_RAW_cal__sam_", 149="IDS0355_210906_RAW_cal__sam_", 150="IDS0369_210908_RAW_cal__sam_", 151="IDS0387_210910_RAW_cal__sam_", 152="IDS0417_220525_RAW_cal__sam_", 153="IDS0168_210310_RAW_cal__sam_", 154="IDS0219_210310_RAW_cal__sam_", 155="IDS0193_210310_RAW_cal__sam_", 156="IDS0418_220525_RAW_cal__sam_", 157="IDS0435_220527_RAW_cal__sam_", 158="IDS0452_220528_RAW_cal__sam_", 159="IDS0469_220530_RAW_cal__sam_", 160="IDS0488_220602_RAW_cal__sam_", 161="IDS0294_210427_RAW_cal__sam_", 162="IDS0321_210901_RAW_cal__sam_", 163="IDS0370_210908_RAW_cal__sam_", 164="IDS0388_210910_RAW_cal__sam_", 165="IDS0169_210310_RAW_cal__sam_", 166="IDS0391_210910_RAW_cal__sam_", 167="IDS0439_220527_RAW_cal__sam_", 168="IDS0395_210910_RAW_cal__sam_", 169="IDS0392_210910_RAW_cal__sam_", 170="IDS0389_210910_RAW_cal__sam_", 171="IDS0218_210310_RAW_cal__sam_", 172="IDS0453_220529_RAW_cal__sam_", 173="IDS0194_210310_RAW_cal__sam_", 174="IDS0293_210427_RAW_cal__sam_", 175="IDS0322_210901_RAW_cal__sam_", 176="IDS0371_210908_RAW_cal__sam_", 177="IDS0390_210910_RAW_cal__sam_", 178="IDS0419_220525_RAW_cal__sam_", 179="IDS0436_220527_RAW_cal__sam_", 180="IDS0454_220529_RAW_cal__sam_", 181="IDS0470_220530_RAW_cal__sam_", 182="IDS0489_220602_RAW_cal__sam_", 183="IDS0170_210310_RAW_cal__sam_", 184="IDS0420_220525_RAW_cal__sam_", 185="IDS0421_220525_RAW_cal__sam_", 186="IDS0471_220530_RAW_cal__sam_", 187="IDS0195_210310_RAW_cal__sam_", 188="IDS0472_220530_RAW_cal__sam_", 189="IDS0306_210831_RAW_cal__sam_", 190="IDS0323_210901_RAW_cal__sam_", 191="IDS0422_220525_RAW_cal__sam_", 192="IDS0437_220527_RAW_cal__sam_", 193="IDS0455_220529_RAW_cal__sam_", 194="IDS0490_220602_RAW_cal__sam_", 195="IDS0372_210908_RAW_cal__sam_", 196="IDS0393_210910_RAW_cal__sam_", 197="IDS0171_210310_RAW_cal__sam_", 198="IDS0196_210310_RAW_cal__sam_", 199="IDS0324_210901_RAW_cal__sam_", 200="IDS0438_220527_RAW_cal__sam_", 201="IDS0456_220529_RAW_cal__sam_", 202="IDS0473_220531_RAW_cal__sam_", 203="IDS0373_210908_RAW_cal__sam_", 204="IDS0394_210910_RAW_cal__sam_", 205="IDS0172_210310_RAW_cal__sam_"}
  out "constrained filename lookup":map{i32, string}(c390)={0="IDS0442_220528_RAW_cal__ref_", 1="IDS0210_210310_RAW_cal__ref_", 2="IDS0443_220528_RAW_cal__ref_", 3="IDS0444_220528_RAW_cal__ref_", 4="IDS0441_220527_RAW_cal__ref_", 5="IDS0445_220528_RAW_cal__ref_", 6="IDS0446_220528_RAW_cal__ref_", 7="IDS0447_220528_RAW_cal__ref_", 8="IDS0448_220528_RAW_cal__ref_", 9="IDS0449_220528_RAW_cal__ref_", 10="IDS0450_220528_RAW_cal__ref_", 11="IDS0451_220528_RAW_cal__ref_", 12="IDS0452_220528_RAW_cal__ref_", 13="IDS0453_220529_RAW_cal__ref_", 14="IDS0454_220529_RAW_cal__ref_", 15="IDS0455_220529_RAW_cal__ref_", 16="IDS0456_220529_RAW_cal__ref_"}
  out "mathematica thing":map{string, map{T2, dbl}}(c390)
  out "temps&degs":map{string, map{T2, dbl}}(c390)
  out "all short filenames":map{string, string}(c390)
  out "all full filenames":map{string, path}(c390)
  out "data file parameters map":map{T2, T18}(c390)
  out "side map to NUM":map{T8, i32}(c390)={enum."sam"=8000, enum."ref"=4000}
  out "side map to STR":map{T8, string}(c390)={enum."sam"="_sam_", enum."ref"="_ref_"}
  out "side map from NUM":map{i32, T8}(c390)={4000=enum."ref", 8000=enum."sam"}
  in  "reverse cursor index map":map{i32, T2}(c390)
  out "state of all selectors":map{T2, map{bool, dbl}}(c390)
  out "state of all selectors string":string="__6.0T__0.0deg__4000side_"
  out "new selector names":map{T2, map{T19, string}}(c390)
  in  "cursor index map":map{T2, i32}(c390)
  in  "load & stuff tab 3":enum32{"Page 2"}(tab)
  in  "load & stuff tab 2":enum32{"Page 2"}(tab)
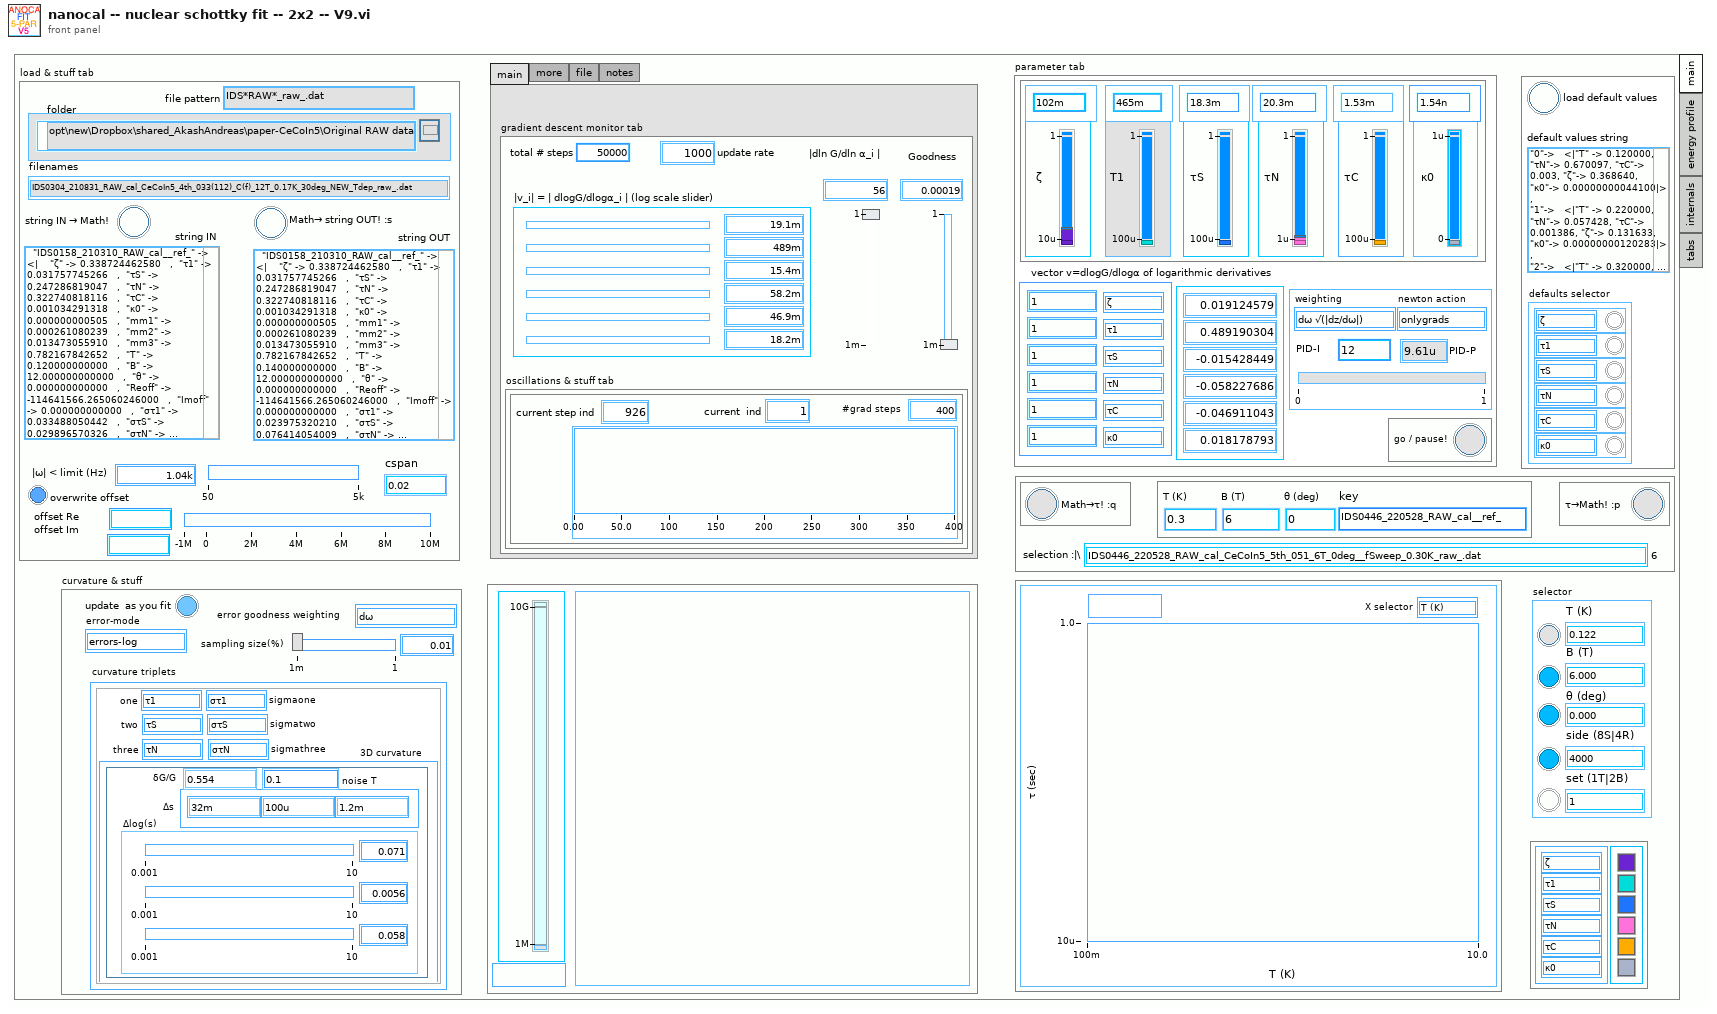
[diagram p1: front panel]
types:
  T1 = enum32{"main", "energy profile", "internals", "tabs"}
  T2 = typedef "3-lorentzian-parameters.ctl" = enum16{"ζ", "τ1", "τS", "τN", "τC", "κ0", "m1", "m2", "m3", "T (K)", "B (T)", "θ (deg)", "side (S|R)", "set of (B|T)", "Re(offset)", "Im(offset)", "στ1", "στ1-", "στ1+", "στS", "στS-", "στS+", "στN", "στN-", "στN+", "τ11", "τ12", "τ21", "τ22", "τN1", "τN2"}
  T3 = typedef "nanocal -- gradient descent -- parameters.ctl" = cluster{"newton action":T4, "weighting":T5, "PID-P":dbl, "PID-I":i32}
  T4 = typedef "3-lorentzian-heat-response action.ctl" = enum16{"calc R", "create string", "calc m1m2m3", "dζ", "dT1", "dτS", "dτN", "dτC", "d-all", "dκ0", "T(K)", "m1", "m2", "m3", "parse string", "θ (deg)", "B (T)", "onlygrads", "newton", "create emty string"}
  T5 = typedef "nanocal-goodness-weighting-strategy.ctl" = enum16{"dω", "dω √(|dz/dω|)", "dω |dz/dω|", "phase", "andreas", "sum", "1/f noise"}
  T6 = typedef "nanocal_data_read_format.ctl" = enum16{"as is", "add - ω", "full rydh", "raw nanocal"}
  T7 = typedef "filename-pattern.ctl" = cluster{"prefix":string, "group":string}
  T8 = typedef "nanocal_side_selector.ctl" = enum16{"sam", "ref"}
  T9 = cluster{"Plost: sweep window":T2, "used default":bool}[]
  T10 = cluster{"ignore set of !":bool, "set (1T|2B)":i32, "ignore side !":bool, "side (8S|4R)":i32, "ignore θ !":bool, "ignore B !":bool, "T (K)":u16, "ignore T !":bool, "θ (deg)":u16, "B (T)":u16, "lookup":cluster{"set of lookup":map{i32, dbl}, "all set of":set{dbl}, "T lookup":map{i32, dbl}, "θ lookup":map{i32, dbl}, "B lookup":map{i32, dbl}, "all T's":set{dbl}, "all θ's":set{dbl}, "all B's":set{dbl}, "all sides":set{dbl}, "side lookup":map{i32, dbl}}}
  T11 = typedef "3D curvature triplet control.ctl" = cluster{"one":T2, "two":T2, "sigmaone":T2, "sigmatwo":T2, "3D curvature":T12, "three":T2, "sigmathree":T2, "pars & errors":map{T2, dbl}}
  T12 = typedef "3D curvature tensor.ctl" = cluster{"curvature Matrix":T13, "eigenvs":dbl[], "Eigenvectors":T14, "theta (rad)":dbl, "theta (deg)":dbl, "Δs":dbl[], "δG/G":dbl, "Δlog(s)":dbl[], "inverse Matrix":T13, "noise T":dbl}
  T13 = typedef "NI_Matrix.lvlib/RealMatrix.ctl" = dbl[][]
  T14 = typedef "NI_Matrix.lvlib/ComplexMatrix.ctl" = cdb[][]
  T15 = typedef "nanocal generate curvature ellipse -- action.ctl" = enum16{"errors-log", "errors-linear"}
  T16 = typedef "show-win- control.ctl" = cluster{"cen (Hz)":dbl, "win (Hz)":dbl, "left (Hz)":dbl, "right (Hz)":dbl}
  T17 = typedef "cursor winow.ctl" = cluster{"left":dbl, "right ":dbl, "center":dbl, "window":dbl, "cursors":i32[], "relative":i32, "absolute":i32, "fixed vertical offset":dbl, "vertical offset":dbl, "skew":dbl, "default window frac":dbl, "kind":enum16{"symmetric", "skewed", "fancy"}, "skew.left":dbl, "skew.right":dbl, "Plot ref":refnum<vi>, "wing order":enum16{"forw", "back"}}
  T18 = typedef "filename-action.ctl" = enum16{"rewrite", "parse", "force pattern", "uniquenum", "get T", "get B", "get ind", "get deg", "get name", "get folder", "get extension", "get basename", "get side", "get setof", "getID", "getIDStock"}
  T19 = typedef "nameformattingitem.ctl" = enum16{"name", "nameL", "units", "prec"}
  T20 = cluster{"keys":T2[], "regexps":string[], "labels":string[]}
  T21 = typedef "cursor action.ctl" = enum16{"range", "read", "write", "check", "zoom out", "smart zoom out", "zoom to aspect ratio 1", "zoom to win", "zoom out 20%", "zoom in 20%", "-empty", "smart zoom out&aspect", "move range left 20%", "move range right 20%", "move range up 20%", "move range down 20%", "zoom to X win", "zoom to Y win", "zoom out X", "zoom out Y", "zoom in X", "zoom in Y", "check plot scale", "set plot color", "set Xlabel", "set Ylabel", "set cursor color"}
  T22 = typedef "cursor window action.ctl" = enum16{"balance", "h. offset change", "cursor moves", "change center", "change window", "init", "check", "reset", "set y to middle", "idle", "-write all Y", "-write left.X", "-write center.X", "-write right.X", "-write all X", "-change center", "-change window", "-change skew", "-read cursor 2", "-read cursor 1", "-read cursor 0", "-read all cursors", "-reset", "-read plot scale", "-set y to middle", "-Q: center.Y is visible", "-Q: window is visible", "-parse center.Y", "-right left from center", "-left move", "-right move", "-set center.Y", "-empty", "-set cursors to default", "-check", "-write center.Y", "-copy cursor 1", "-copy cursor 0", "-copy cursor 2", "move right", "move left", "shrink", "broaden", "skew up", "skew down", "-write plot scale", "zoom X", "change cen&win", "zoom to all data", "color--red", "color--green", "color--yellow", "read", "zoom out", "zoom in", "slide right", "slide left", "set range aspect ratio to 1", "move to window range", "--move to window range"}
  T23 = typedef "publisher action.ctl" = enum16{"set", "get", "init", "check"}
  T24 = typedef "nanocal -- gradient descent -- action.ctl" = enum16{"init", "step", "peek"}
  T25 = typedef "cursor sate.ctl" = enum16{"normal", "alert", "fuzzy", "interesting", "boring", "colored"}
  T26 = typedef "mathematica string map action.ctl" = enum16{"create string", "calc m1m2m3", "parse string"}
  T27 = typedef "LVMapReplaceAction.ctl" = enum32{"Modify Entry only if found", "Add or Modify Entry", "Delete Entry"}
  T28 = typedef "nanocal -- defaut parameter manager action-- V1.ctl" = enum16{"get logarithmic interp", "update", "get linear interp"}
  T29 = typedef "nanocal -- plotstring file action.ctl" = enum16{"generate plotstring file", "generate plotstring thing", ""}
  T30 = typedef "file -- read-write control.ctl" = enum16{"read", "write all", "append one line"}
  T31 = typedef "nanocal_raw_file_manage_action_V1.ctl" = enum16{"read S side", "read R side", "read meta", "read_names"}
  T32 = typedef "array -- freq-voltage transformations action.ctl" = enum16{"as is", "add -ω", "sort ω", "2 x ω", "R-phase(deg) to Re-Im", "select ω>0", "labview file str", "select |ω|<max"}
  T33 = typedef "KM_file -- read-write control.ctl" = enum16{"read", "write all", "append one line"}
  T34 = typedef "nanocal -- gradient descent-- data.ctl" = cluster{"dz/dω  (sec/rad)":cdb[], "z ":cdb[], "ω (rad/sec)":dbl[]}
  T35 = typedef "array action.ctl" = enum16{"generate range", "generate log range"}
  T36 = typedef "LVRangeTypeDef.ctl" = cluster{"Minimum":dbl, "Maximum":dbl, "Increment":dbl, "Minor Increment":dbl, "Start":dbl}
  T37 = typedef "2Dwindow.ctl" = cluster{"window y":dbl, "center x":dbl, "center y":dbl, "window x":dbl}
  T38 = typedef "eventvkey.ctl" = enum16{"ASCII", "Enter", "Return", "Shift", "Ctrl", "Alt", "Cmd", "Opt", "Caps", "NumLock", "Clear", "Break", "Up", "Down", "Left", "Right", "Insert", "Delete", "Home", "End", "PageUp", "PageDown", "Escape", "Help", "Pause", "ScrollLock", "F1", "F2", "F3", "F4", "F5", "F6", "F7", "F8", "F9", "F10", "F11", "F12", "F13", "F14", "F15", "F16", "F17", "F18", "F19", "F20", "F21", "F22", "F23", "F24", "Play", "VolumeUp", "VolumeDown", "Mute", "Two Byte Char"}
